vi "user32.SetForegroundWindow.vi"(8 "error in":errorcluster caption="error in (no error)", 9 "hWnd":u32) -> (0 "error out":errorcluster, 1 "hWnd out":u32)   [LabVIEW 2018]
uses:
  User32.dll
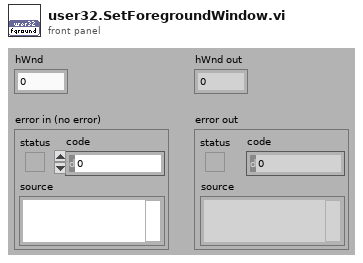
[diagram p1: front panel]
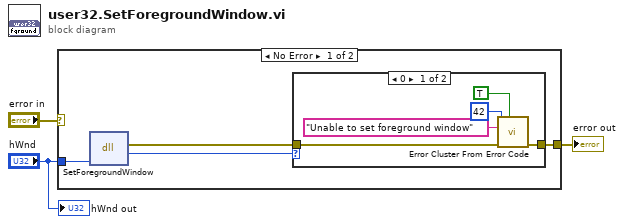
[diagram p0: block diagram]
diagram:
  n1 = case shown="No Error" "error in" {
    selector: "error in" -> [_ w14]
    tunnel: [w7 w14] -> w2
    tunnel: "hWnd" -> [w6 _]
    frame No Error {
      n2 = dll-call lib="USER32.DLL" fn="SetForegroundWindow"("hwnd"=w6) -> (error out=w4:errorcluster, "return"=w5:u32)  [unwired: 4 in, 1 out]
      n3 = case shown="0" w5 {
        tunnel: [w12 w13] -> w7
        tunnel: w4 -> [w10 w13]
        frame 0 {
          n4 = call <vilib>:"Error Cluster From Error Code.vi"("show call chain? (False)"=TRUE, "error in (no error)"=w10, "error message (\"\")"="Unable to set foreground window" ("format string"), "error code (0)"=42) -> ("error out"=w12:errorcluster)  [unwired: 5 in]
        }
        frame Default {
        }
      }
    }
    frame Error {
    }
  }
  "error out" <- w2
  "hWnd out" <- "hWnd"
